vi "Check State Transitions.vi"(8 "error in (no error)":refnum<class "MultiErrors.lvclass">, 11 "Sequence Validation in":refnum<class "Sequence Validation.lvclass">) -> (0 "error out":refnum<class "MultiErrors.lvclass">, 3 "Sequence Validation out":refnum<class "Sequence Validation.lvclass">)   [LabVIEW 2020, in "VolatusSeq.lvlib" / "Sequence Validation.lvclass"]
uses:
  Sequence Validation.lvclass
  Sequence Validation.lvclass/Sequence Validation.ctl
  Sequence Config/Sequence Config.lvclass
  VolatusErrorUtilities/MultiErrors/MultiErrors.lvclass
  State Transition Config/State Transition Config.lvclass
  Transition Config/Transition Config.lvclass
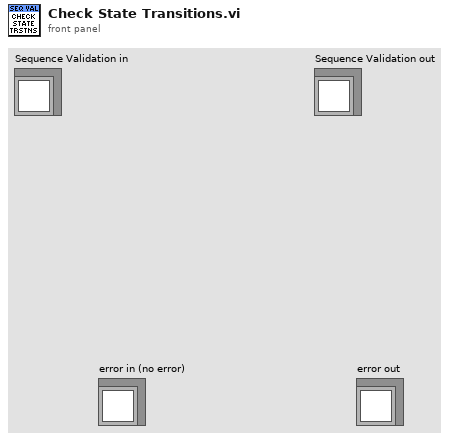
[diagram p1: front panel]
types:
  T1 = typedef "VolatusSeqConfig.lvlib/State.ctl" = cluster{"Name":string, "Steps":T2[], "Transitions":refnum<class "Transition Config.lvclass">[], "Comment":string, "Color":string}
  T2 = typedef "VolatusSeqConfig.lvlib/Step.ctl" = cluster{"Time":dbl, "Commands":refnum<class "Command Config.lvclass">[]}
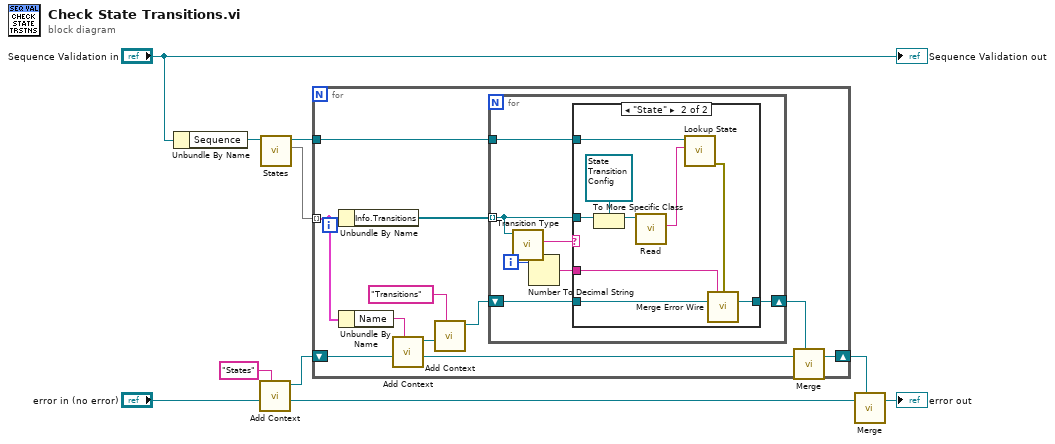
[diagram p0: block diagram]
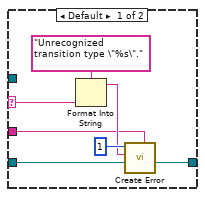
[diagram p2: hidden frame]
diagram:
  n1 = Unbundle By Name("Sequence Validation in") -> ("Sequence"=w8:refnum<class "Sequence Config.lvclass">)
  n2 = call "Add Context.vi"("Context"="States", "MultiErrors in"="error in (no error)") -> ("Original Context"=w7:refnum<class "MultiErrors.lvclass">, "Added Context"=w5:refnum<class "MultiErrors.lvclass">)  [unwired: 8 in]
  n3 = call "States.vi"("Sequence Config in"=w8) -> ("States"=w4:map{string, T1}, "Sequence Config out"=w1:refnum<class "Sequence Config.lvclass">)  [unwired: 8 in, 1 out]
  n4 = for {
    shift-right: [w12] -> w2
    shift-left: w5 -> [w21]
    tunnel: w4 -> [w19] mode=indexing
    tunnel: w1 -> [w11]
    n5 = Unbundle By Name(w19) -> ("Info.Transitions"=w18:refnum<class "Transition Config.lvclass">[])
    n6 = Unbundle By Name(w19) -> ("Name"=w20:string)
    n7 = call "Add Context.vi"("Context"=w20, "MultiErrors in"=w21) -> ("Original Context"=w14:refnum<class "MultiErrors.lvclass">, "Added Context"=w17:refnum<class "MultiErrors.lvclass">)  [unwired: 8 in]
    n8 = call "Add Context.vi"("Context"="Transitions", "MultiErrors in"=w17) -> ("Added Context"=w15:refnum<class "MultiErrors.lvclass">)  [unwired: 8 in, 1 out]
    n9 = for {
      shift-right: [w26] -> w13
      shift-left: w15 -> [w27]
      tunnel: w18 -> [w25] mode=indexing
      tunnel: w11 -> [w24]
      i -> [w23]
      n10 = call-dynamic "Transition Type.vi"("Transition Config in"=w25) -> ("Transition Type"=w28:string)  [unwired: 10 in]
      n11 = Number To Decimal String(number=w23) -> (decimal integer string=w22:string)  [unwired: 1 in]
      n12 = case shown="\"State\"" w28 {
        selector: w28 -> [w35 _]
        tunnel: w27 -> [w33 w39]
        tunnel: [w30 w37] -> w26
        tunnel: w25 -> [_ w44]
        tunnel: w24 -> [_ w41]
        tunnel: w22 -> [w29 w36]
        frame Default {
          n13 = Format Into String(format string="Unrecognized transition type \"%s\".", w35) -> (resulting string=w31:string)  [unwired: 2 in, 1 out]
          n14 = call "Create Error.vi"("Local Context (None)"=w29, "MultiErrors in"=w33, "Message"=w31, "Code"=1) -> ("MultiErrors out"=w30:refnum<class "MultiErrors.lvclass">)  [unwired: 7 in]
        }
        frame "State" {
          n15 = To More Specific Class(target class=refnum<class "State Transition Config.lvclass"> refnum ("VolatusSeqConfig.lvlib:State Transition Config.lvclass"), reference=w44) -> (specific class reference=w42:refnum<class "State Transition Config.lvclass">)  [unwired: 1 in, 1 out]
          n16 = call "Read.vi"("State Transition Config in"=w42) -> ("Target State"=w40:string)  [unwired: 10 in]
          n17 = call "Lookup State.vi"("State"=w40, "Sequence Config in"=w41) -> ("error out"=w38:errorcluster)  [unwired: 7 in, 2 out]
          n18 = call "Merge Error Wire.vi"("Local Context (None)"=w36, "error in (no error)"=w38, "MultiErrors in"=w39) -> ("MultiErrors out"=w37:refnum<class "MultiErrors.lvclass">)  [unwired: 12 in]
        }
      }
    }
    n19 = call "Merge.vi"("First Error In"=w14, "Second Error In"=w13) -> ("MultiErrors out"=w12:refnum<class "MultiErrors.lvclass">)  [unwired: 5 in]
  }
  n20 = call "Merge.vi"("First Error In"=w7, "Second Error In"=w2) -> ("MultiErrors out"=→"error out":refnum<class "MultiErrors.lvclass">)  [unwired: 5 in]
  "Sequence Validation out" <- "Sequence Validation in"
